vi "Match GLOB.vi"(8 "error in (no error)":errorcluster, 9 "glob":string, 10 "string":string) -> (0 "error out":errorcluster, 2 "match?":bool)   [LabVIEW 2014, in "SQLite3LV.lvlib" / "sqlite3.lvclass"]
doc: "int SQLite3LV Connection_strglob(const char *zGlob, const char *zStr);\n\nThe sqlite3_strglob(P,X) interface returns zero if string X matches the glob pattern P, and it returns non-zero if string X does not match the glob pattern P. The definition of glob pattern matching used in sqlite3_strglob(P,X) is the same as for the \"X GLOB P\" operator in the SQL dialect used by SQLite. The sqlite3_strglob(P,X) function is case sensitive.\n\nNote that this routine returns zero on a match and non-zero if the strings do not match, the same as sqlite3_stricmp() and sqlite3_strnicmp().\n\nSee also lists of Objects, Constants, and Functions."
uses:
  sqlite3.lvclass
  sqlite3_64.dll
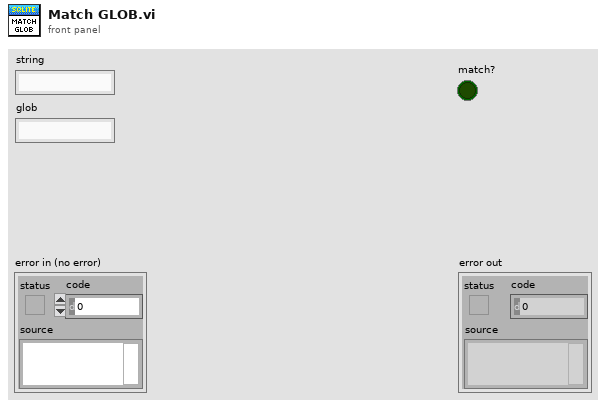
[diagram p1: front panel]
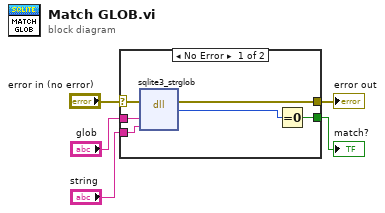
[diagram p0: block diagram]
diagram:
  n1 = case shown="No Error" "error in (no error)" {
    selector: "error in (no error)" -> [w9 w12]
    tunnel: [w8 w12] -> w4
    tunnel: "string" -> [w11 _]
    tunnel: "glob" -> [w10 _]
    tunnel: [w6 _] -> w1
    frame No Error {
      n2 = dll-call lib="C:/Users/BobUser/Desktop/LVTables/sqlite3**.*" fn="sqlite3_strglob"(error in=w9, "pzGlob"=w10, "pzStr"=w11) -> (error out=w8:errorcluster, "result"=w7:i32)  [unwired: 4 in, 1 out]
      n3 = Equal To 0?(x=w7) -> (x = 0?=w6:bool)
    }
    frame Error {
    }
  }
  "error out" <- w4
  "match?" <- w1
